vi "Clear Volumes.vi"(8 "error in (no error)":errorcluster, 11 "PHD Ultra in":refnum<class "cetoni.lvclass">) -> (0 "error out":errorcluster, 3 "PHD Ultra out":refnum<class "cetoni.lvclass">)   [LabVIEW 2018, in "cetoni.lvlib" / "cetoni.lvclass"]
uses:
  cetoni.lvclass
  cetoni.lvclass/cetoni.ctl
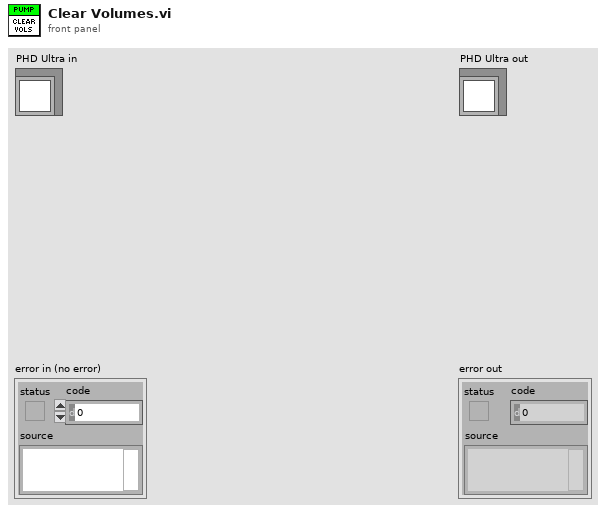
[diagram p1: front panel]
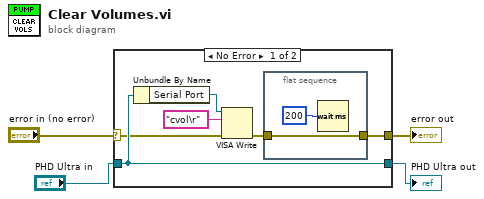
[diagram p0: block diagram]
diagram:
  n1 = case shown="No Error" "error in (no error)" {
    selector: "error in (no error)" -> [w7 w14]
    tunnel: [w5 w14] -> w3
    tunnel: [w9 w13] -> w1
    tunnel: "PHD Ultra in" -> [w9 w13]
    frame No Error {
      n2 = Unbundle By Name(w9) -> ("Serial Port"=w8:refnum<visa-resource-name>)
      n3 = VISA Write(VISA resource name=w8, write buffer="cvol\r", error in (no error)=w7) -> (error out=w6:errorcluster)  [unwired: 2 out]
      n4 = flat-sequence {
        tunnel: w6 -> [w12]
        tunnel: [w12] -> w5
        frame #0 {
          n5 = Wait (ms)(milliseconds to wait=u32 200) -> ()  [unwired: 1 out]
        }
      }
    }
    frame Error {
    }
  }
  "error out" <- w3
  "PHD Ultra out" <- w1
